vi "Path_Filter.vi"(0 "path":path, 11 "error in":errorcluster) -> (4 "File/Folder Name":string, 6 "Size":string, 15 "error out":errorcluster)   [LabVIEW 2023, in "Unit Testing CA1.lvlib"]
uses:
  Unit Testing CA1.lvlib
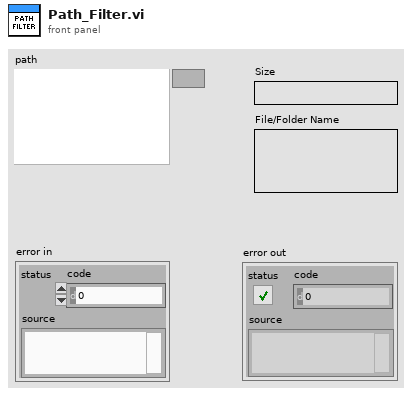
[diagram p1: front panel]
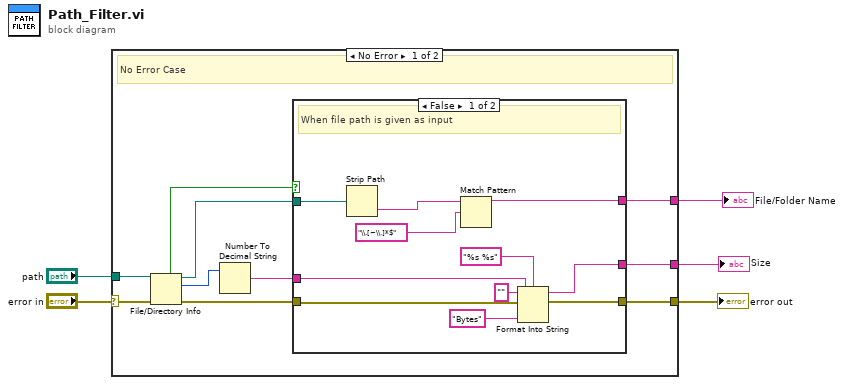
[diagram p0: block diagram]
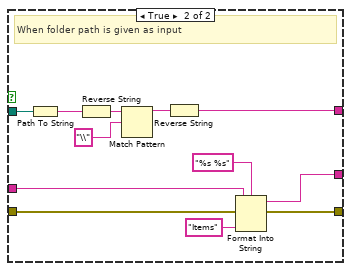
[diagram p2: hidden frame]
diagram:
  n1 = case shown="No Error" "error in" {
    selector: "error in" -> [w15 w39]
    tunnel: [w6 w39] -> w4
    tunnel: "path" -> [w10 _]
    tunnel: [w9 _] -> w2
    tunnel: [w8 _] -> w1
    frame No Error {
      # "No Error Case"
      n2 = File/Directory Info(path=w10, error in=w15) -> (path out=w13:path, directory=w14:bool, size=w12:i64, error out=w7:errorcluster)  [unwired: 3 out]
      n3 = Number To Decimal String(number=w12) -> (decimal integer string=w11:string)  [unwired: 1 in]
      n4 = case shown="False" w14 {
        tunnel: w13 -> [w24 w38]
        tunnel: [w23 w34] -> w8
        tunnel: w11 -> [w20 w31]
        tunnel: [w19 w29] -> w9
        tunnel: w7 -> [w18 w28]
        tunnel: [w17 w27] -> w6
        frame False {
          # "When file path is given as input"
          n5 = Strip Path(path=w24) -> (name=w26:string)  [unwired: 1 out]
          n6 = Match Pattern(string=w26, regular expression="\\.[~\\.]*$") -> (before substring=w23:string)  [unwired: 4 out]
          n7 = Format Into String(format string="%s %s", initial string="", error in=w18, w20, "Bytes" ("input 2")) -> (resulting string=w19:string, error out=w17:errorcluster)
        }
        frame True {
          # "When folder path is given as input"
          n8 = Path To String(path=w38) -> (string=w37:string)
          n9 = Reverse String(1:w37) -> (0:w36:string)
          n10 = Match Pattern(string=w36, regular expression="\\") -> (before substring=w35:string)  [unwired: 1 in, 3 out]
          n11 = Reverse String(1:w35) -> (0:w34:string)
          n12 = Format Into String(format string="%s %s", error in=w28, w31, "Items" ("input 2")) -> (resulting string=w29:string, error out=w27:errorcluster)  [unwired: 1 in]
        }
      }
    }
    frame Error {
    }
  }
  "error out" <- w4
  "File/Folder Name" <- w1
  "Size" <- w2
